vi "sequence2.vi"() -> ()   [LabVIEW 2021]
panel:
  out "Array 2":string[](array[string])
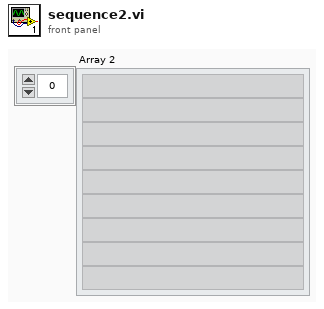
[diagram p1: front panel]
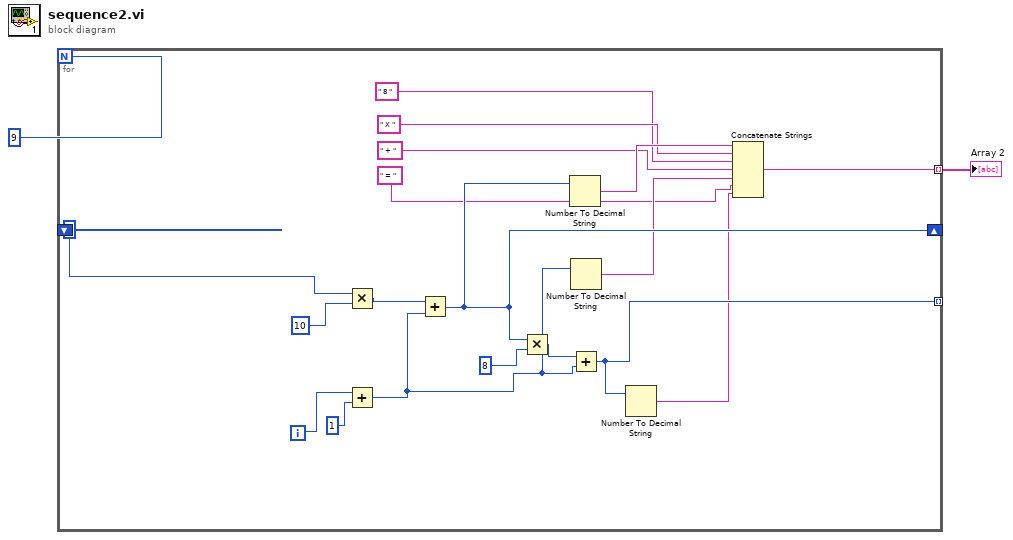
[diagram p0: block diagram]
diagram:
  n1 = for {
    N: 9 -> [_]
    shift-right: [w14] -> _
    shift-left: 0 -> [w21]
    tunnel: [w13] -> _ mode=indexing
    tunnel: [w4] -> w1 mode=indexing
    i -> [w19]
    n2 = Multiply(x=w21, y=10) -> (x*y=w17:i32)
    n3 = Add(x=w19, y=1) -> (x+y=w8:i32)
    n4 = Add(x=w17, y=w8) -> (x+y=w14:i32)
    n5 = Multiply(x=w14, y=8) -> (x*y=w15:i32)
    n6 = Number To Decimal String(number=w14) -> (decimal integer string=w12:string)  [unwired: 1 in]
    n7 = Number To Decimal String(number=w8) -> (decimal integer string=w7:string)  [unwired: 1 in]
    n8 = Add(x=w15, y=w8) -> (x+y=w13:i32)
    n9 = Number To Decimal String(number=w13) -> (decimal integer string=w5:string)  [unwired: 1 in]
    n10 = Concatenate Strings(w12, " X ", " 8 ", " + ", w7, " = ", w5) -> (w4:string)
  }
  "Array 2" <- w1
